vi "Overlay.vi"(8 "error in (no error)":errorcluster, 10 "Image In":T1, 11 "Overlay Base in":refnum<class "Analyze Results Total Counts.lvclass">) -> (0 "error out":errorcluster, 2 "Image out":T1, 3 "Overlay Base out":refnum<class "Analyze Results Total Counts.lvclass">)   [LabVIEW 2020, in "Analyze Results Total Counts.lvclass"]
uses:
  Analyze Results Total Counts.lvclass
  C:/POLARIS Programme/POLARIS-AS-3-Cams/Submodules/HIJ Vision/Analyze/Results and Overlays/Results Base/Analyze Results Base.lvclass
  <vilib>/vision/Image Controls.llb/IMAQ Image.ctl
  Analyze Results Total Counts.lvclass/Analyze Results Total Counts.ctl
  Results Base/Analyze Results Base.lvclass/Analyze Results Base.ctl
  Read Total Counts.vi
  Results Base/Read Font, Size & Style.vi
  Results Base/Read Position.vi
  Results Base/Read Overlay colors.vi
  Results Base/Read Overlay_.vi
  Results Base/Analyze Results Base.lvclass
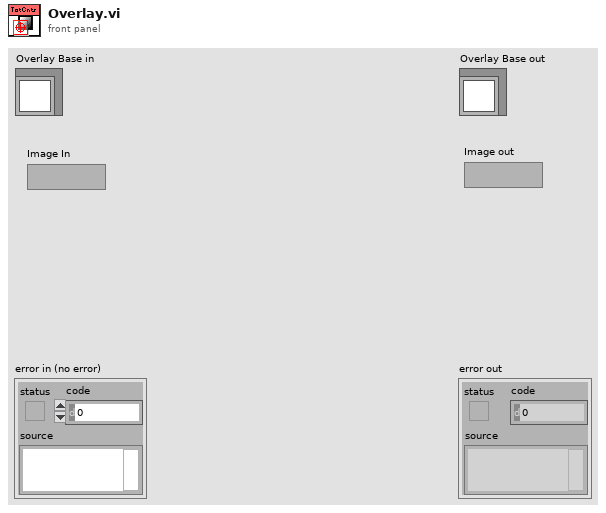
[diagram p1: front panel]
types:
  T1 = typedef "IMAQ Image.ctl" = refnum<image>
  T2 = cluster{"Desired Font (Application)":enum16{"User-specified Font", "Application Font", "System Font", "Dialog Font"}, "[User-specified Font]":cluster{"Font Name":string, "Size":i16, "Strikeout?":bool, "Italic?":bool, "Underline?":bool, "Outline?":bool, "Shadow?":bool, "Bold?":bool, "Rotation Angle":dbl}, "Horizontal Alignment":i16, "Vertical Alignment":i16}
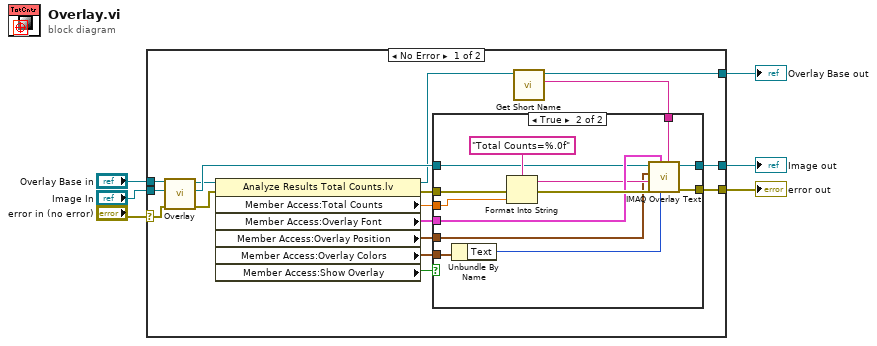
[diagram p0: block diagram]
diagram:
  n1 = case shown="No Error" "error in (no error)" {
    selector: "error in (no error)" -> [w9 w41]
    tunnel: "Overlay Base in" -> [w19 w40]
    tunnel: "Image In" -> [w18 w39]
    tunnel: [w8 w40] -> w4
    tunnel: [w16 w39] -> w3
    tunnel: [w13 w41] -> w2
    frame No Error {
      n2 = call-parent "Overlay.vi"("error in (no error)"=w9, "Image In"=w18, "Overlay Base in"=w19) -> ("error out"=w21:errorcluster, "Image out"=w23:T1, "Overlay Base out"=w20:refnum<class "Analyze Results Total Counts.lvclass">)  [unwired: 6 in]
      n3 = property class="Analyze Results Total Counts.lv"(reference=w20, error in=w21) -> (reference out=w17:refnum<class "Analyze Results Total Counts.lvclass">, error out=w22:errorcluster, "Member Access:Total Counts"=w15:dbl, "Member Access:Overlay Font"=w10:T2, "Member Access:Overlay Position"=w14:cluster{"x":i16, "y":i16}, "Member Access:Overlay Colors"=w12:cluster{"Border":u32, "Text":u32}, "Member Access:Show Overlay"=w11:bool)
      n4 = call-dynamic "Get Short Name.vi"("Analyze Results Base in"=w17) -> ("Short Name"=w7:string, "Analyze Results Base out"=w8:refnum<class "Analyze Results Total Counts.lvclass">)  [unwired: 8 in, 1 out]
      n5 = case shown="True" w11 {
        tunnel: w23 -> [w25 w31]
        tunnel: [w25 w34] -> w16
        tunnel: w22 -> [w24 w30]
        tunnel: [w24 w33] -> w13
        tunnel: w10 -> [_ w36]
        tunnel: w15 -> [_ w29]
        tunnel: w14 -> [_ w28]
        tunnel: w12 -> [_ w27]
        tunnel: w7 -> [_ w26]
        frame False {
        }
        frame True {
          n6 = Unbundle By Name(w27) -> ("Text"=w32:u32)
          n7 = Format Into String(format string="Total Counts=%.0f", error in=w30, w29) -> (resulting string=w35:string, error out=w37:errorcluster)  [unwired: 1 in]
          n8 = call "IMAQ Overlay Text"("Group"=w26, "Text Color (black)"=w32, "Font, Size & Style"=w36, "error in (no error)"=w37, "String"=w35, "Origin"=w28, "Image"=w31) -> ("error out"=w33:errorcluster, "Image Out"=w34:T1)  [unwired: 3 in]
        }
      }
    }
    frame Error {
    }
  }
  "error out" <- w2
  "Overlay Base out" <- w4
  "Image out" <- w3
